vi "Init New Binding.vi"(8 "Motor Labels":string[](array[string]), 9 "Action List":T3(array[cluster]), 10 "TriggerAction Cluster":T2, 11 "Triggers Arr Ref":refnum<vi>) -> (1 "Array of Data Types":T1(array[cluster]), 2 "Array of Data Names&Defaults":cluster{"Data Names&Defaults":string[][]}[](array[cluster]), 3 "2-col Arr Actions out":string[][](array[string]))   [LabVIEW 2016, in "Hardware.lvlib" / "Motions.lvlib" / "Motions.lvclass"]
uses:
  <userlib>/Common Components/Hardware/Abstract System/Motions/Motions/Motions.lvclass
  <userlib>/Common Components/Hardware/Abstract System/Motions/Motions/TA Binding Data.ctl
panel:
  # "Action Name"
  # "Formatted String"
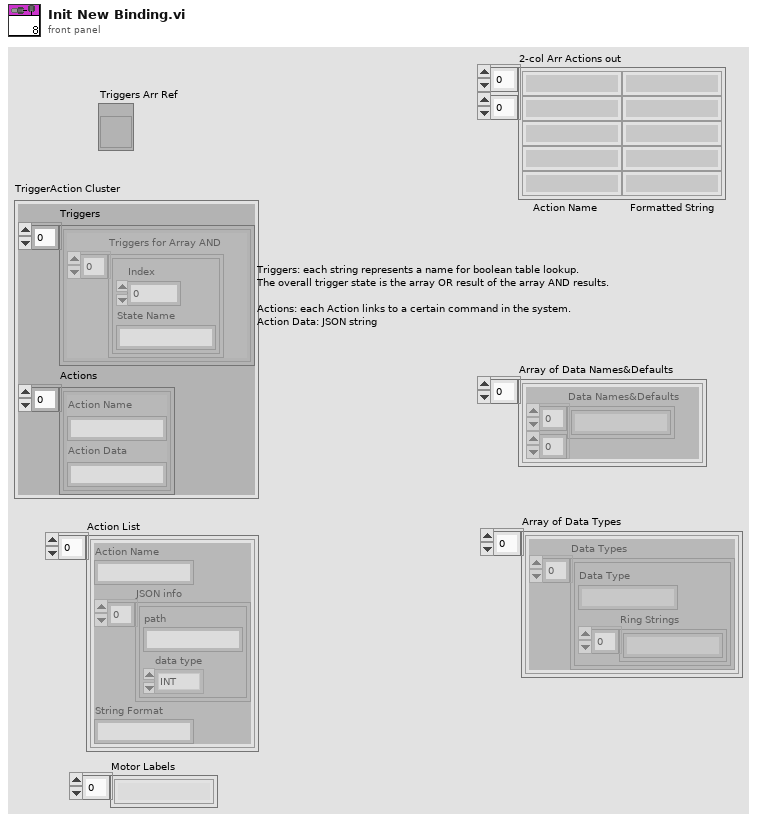
[diagram p1: front panel]
types:
  T1 = cluster{"Data Types":cluster{"Data Type":string, "Ring Strings":string[]}[]}[]
  T2 = typedef "Hardware.lvlib/Motions.lvlib/Motions.lvclass/TA Binding Data.ctl" = cluster{"Triggers":cluster{"Triggers for Array AND":cluster{"Index":u8, "State Name":string}[]}[], "Actions":cluster{"Action Name":string, "Action Data":string}[]}
  T3 = cluster{"Action Name":string, "JSON info":cluster{"path":string, "data type":enum16{"INT", "DBL", "BOOL", "String"}}[], "String Format":string}[]
  T4 = cluster{"Triggers for Array AND":cluster{"Index":u8, "State Name":string}[]}[]
  T5 = cluster{"Action Name":string, "Action Data":string}[]
  T6 = cluster{"Action Name":string, "JSON info":cluster{"path":string, "data type":enum16{"INT", "DBL", "BOOL", "String"}}[], "String Format":string}
  T7 = cluster{"path":string, "data type":enum16{"INT", "DBL", "BOOL", "String"}}[]
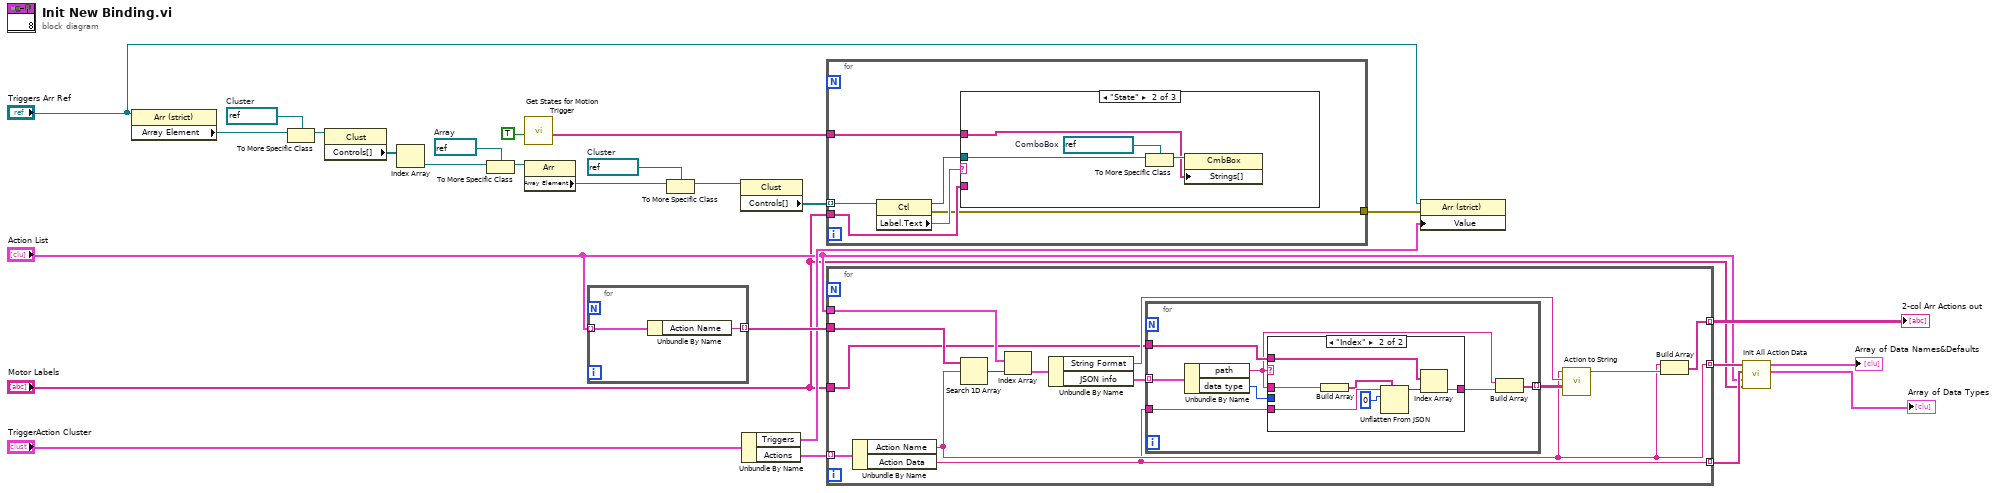
[diagram p0: block diagram]
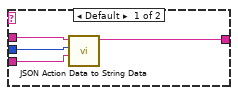
[diagram p2: hidden frame]
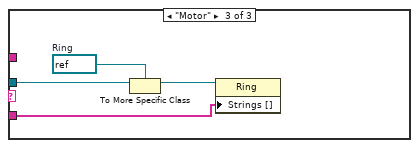
[diagram p4: hidden frame]
diagram:
  w21 = refnum<vi> refnum  # Cluster
  w19 = refnum<vi> refnum  # Array
  w15 = refnum<vi> refnum  # Cluster
  n1 = property on="Property Node" class="Arr (strict)"(reference="Triggers Arr Ref") -> ("Array Element"=w14:refnum<vi>)  [unwired: 1 in, 2 out]
  n2 = To More Specific Class(target class=w15, reference=w14) -> (specific class reference=w16:refnum<vi>)  [unwired: 1 in, 1 out]
  n3 = property class="Clust"(reference=w16) -> ("Controls[]"=w17:refnum<vi>[])  [unwired: 1 in, 2 out]
  n4 = Index Array(array=w17) -> (element=w18:refnum<vi>)  [unwired: 1 in]
  n5 = To More Specific Class(target class=w19, reference=w18) -> (specific class reference=w20:refnum<vi>)  [unwired: 1 in, 1 out]
  n6 = call <userlib>:"Get States for Motion Trigger.vi"("Names only?"=TRUE) -> ("Array of Trigger State Names"=w26:string[])  [unwired: 7 in, 3 out]
  n7 = property class="Arr"(reference=w20) -> ("Array Element"=w22:refnum<vi>)  [unwired: 1 in, 2 out]
  n8 = for {
    tunnel: "Action List" -> [w28] mode=indexing
    tunnel: [w27] -> w12 mode=indexing
    n9 = Unbundle By Name(w28) -> ("Action Name"=w27:string)
  }
  n10 = To More Specific Class(target class=w21, reference=w22) -> (specific class reference=w23:refnum<vi>)  [unwired: 1 in, 1 out]
  n11 = property class="Clust"(reference=w23) -> ("Controls[]"=w24:refnum<vi>[])  [unwired: 1 in, 2 out]
  n12 = Unbundle By Name("TriggerAction Cluster") -> ("Triggers"=w8:T4, "Actions"=w10:T5)
  n13 = for {
    tunnel: w24 -> [w34] mode=indexing
    tunnel: "Motor Labels" -> [w31]
    tunnel: w26 -> [w30]
    tunnel: [w29] -> w7
    n14 = property class="Ctl"(reference=w34) -> (reference out=w32:refnum<vi>, error out=w29:errorcluster, "Label.Text"=w33:string)  [unwired: 1 in]
    n15 = case shown="\"State\"" w33 {
      tunnel: w32 -> [_ w36 w41]
      tunnel: w31 -> [_ _ w39]
      tunnel: w30 -> [_ w35 _]
      frame Default {
      }
      frame "State" {
        w38 = refnum<vi> refnum  # ComboBox
        n16 = To More Specific Class(target class=w38, reference=w36) -> (specific class reference=w37:refnum<vi>)  [unwired: 1 in, 1 out]
        n17 = property class="CmbBox"(reference=w37, "Strings[]"=w35) -> ()  [unwired: 1 in, 2 out]
      }
      frame "Motor" {
        w42 = refnum<vi> refnum  # Ring
        n18 = To More Specific Class(target class=w42, reference=w41) -> (specific class reference=w40:refnum<vi>)  [unwired: 1 in, 1 out]
        n19 = property class="Ring"(reference=w40, "Strings []"=w39) -> ()  [unwired: 1 in, 2 out]
      }
    }
  }
  n20 = for {
    tunnel: w10 -> [w55] mode=indexing
    tunnel: w12 -> [w54]
    tunnel: [w53] -> w13 mode=indexing
    tunnel: "Action List" -> [w52]
    tunnel: "Motor Labels" -> [w46]
    tunnel: [w44] -> w6 mode=indexing
    tunnel: [w43] -> w5 mode=indexing
    n21 = Unbundle By Name(w55) -> ("Action Name"=w44:string, "Action Data"=w43:string)
    n22 = Search 1D Array(1D array=w54, element=w44) -> (index of element=w51:i32)  [unwired: 1 in]
    n23 = Index Array(array=w52, index=w51) -> (element=w50:T6)
    n24 = Unbundle By Name(w50) -> ("String Format"=w49:string, "JSON info"=w48:T7)
    n25 = for {
      tunnel: w48 -> [w61] mode=indexing
      tunnel: w43 -> [w62]
      tunnel: w46 -> [w59]
      tunnel: [w56] -> w45 mode=indexing
      n26 = Unbundle By Name(w61) -> ("path"=w58:string, "data type"=w60:enum16{"INT", "DBL", "BOOL", "String"})
      n27 = case shown="\"Index\"" w58 {
        tunnel: w62 -> [w64 w73]
        tunnel: w58 -> [w66 w72]
        tunnel: w60 -> [w65 _]
        tunnel: [w63 w67] -> w57
        tunnel: w59 -> [_ w68]
        frame Default {
          n28 = call <userlib>:"JSON Action Data to String Data.vi"("Action Data (JSON)"=w64, "data type"=w65, "path"=w66) -> ("String"=w63:string)  [unwired: 7 in, 1 out]
        }
        frame "Index" {
          n29 = Build Array(w72) -> (w71:string[])
          n30 = Unflatten From JSON(path=w71, JSON string=w73, type and defaults=0) -> (value=w69:i32)  [unwired: 4 in, 1 out]
          n31 = Index Array(array=w68, index=w69) -> (element=w67:string)
        }
      }
      n32 = Build Array(w58, w57) -> (w56:string[])
    }
    n33 = call <userlib>:"Action to String.vi"("Action Data"=w45, "String Format"=w49, "Action Name"=w44) -> ("String"=w47:string)  [unwired: 7 in, 1 out]
    n34 = Build Array(w44, w47) -> (w53:string[])
  }
  "2-col Arr Actions out" <- w13
  n35 = property class="Arr (strict)"(reference="Triggers Arr Ref", error in=w7, "Value"=w8) -> ()  [unwired: 2 out]
  n36 = call <userlib>:"Init All Action Data.vi"("Motor Labels"="Motor Labels", "Action List"="Action List", "Array of Action Data (JSON)"=w5, "Action Names"=w6) -> ("Array of Data Types"=→"Array of Data Types":T1, "Array of Data Names&Defaults"=→"Array of Data Names&Defaults":cluster{"Data Names&Defaults":string[][]}[])  [unwired: 6 in]
